vi "Set Format String.vi"(8 "error in (no error)":errorcluster, 10 "Format String":string="%.6f", 11 "Text Log File Specification in":refnum<class "Text Log File Specification.lvclass">) -> (0 "error out":errorcluster, 3 "Text Log File Specification out":refnum<class "Text Log File Specification.lvclass">)   [LabVIEW 2012, in "Waveform Data Logger Shared.lvlib" / "Text Log File Specification.lvclass"]
uses:
  Text Log File Specification.lvclass
  Text Log File Specification.lvclass/Text Log File Specification.ctl
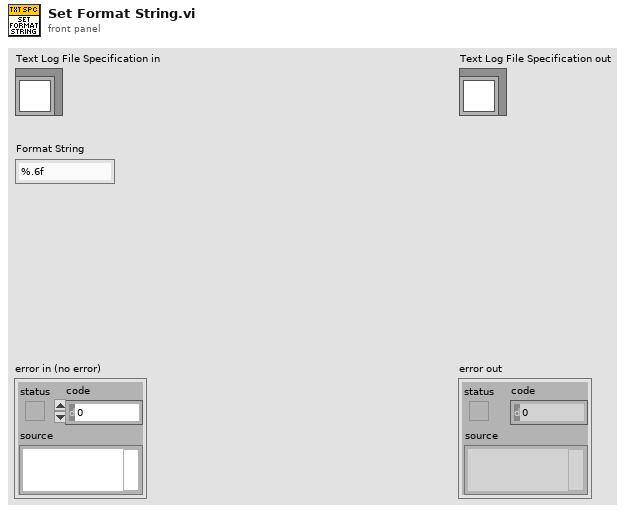
[diagram p1: front panel]
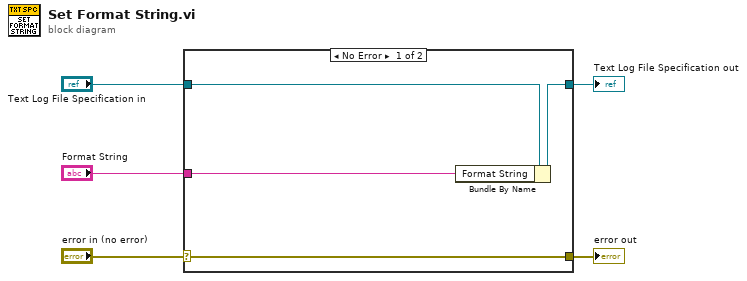
[diagram p0: block diagram]
diagram:
  n1 = case shown="No Error" "error in (no error)" {
    selector: "error in (no error)" -> [w9 w10]
    tunnel: [w9 w10] -> w4
    tunnel: [w7 w11] -> w2
    tunnel: "Text Log File Specification in" -> [w8 w11]
    tunnel: "Format String" -> [w6 _]
    frame No Error {
      n2 = Bundle By Name(cluster=w8, "Format String"=w6) -> (w7:refnum<class "Text Log File Specification.lvclass">)
    }
    frame Error {
    }
  }
  "error out" <- w4
  "Text Log File Specification out" <- w2
